vi "Read Interface.vi"(8 "error in (no error)":errorcluster, 11 "Configuration in":refnum<class "Configuration.lvclass">) -> (0 "error out":errorcluster, 2 "Interface":refnum<class "Interface.lvclass">, 3 "Configuration out":refnum<class "Configuration.lvclass">)   [LabVIEW 2013, in "Configuration.lvlib" / "Configuration.lvclass"]
doc: "Read interface object from class private data.."
uses:
  Configuration.lvclass
  Interface/Interface.lvclass
  Configuration.lvclass/Configuration.ctl
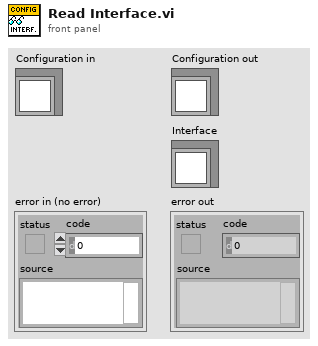
[diagram p1: front panel]
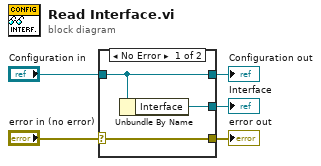
[diagram p0: block diagram]
diagram:
  n1 = case shown="No Error" "error in (no error)" {
    selector: "error in (no error)" -> [w8 w9]
    tunnel: [w8 w9] -> w4
    tunnel: [w7 w10] -> w2
    tunnel: "Configuration in" -> [w7 w10]
    tunnel: [w6 _] -> w1
    frame No Error {
      n2 = Unbundle By Name(w7) -> ("Interface"=w6:refnum<class "Interface.lvclass">)
    }
    frame Error {
    }
  }
  "error out" <- w4
  "Configuration out" <- w2
  "Interface" <- w1
